vi "G#Object_UnregisterObject.vi"(0 "reference in":refnum<class "G#Object.lvclass">, 1 "object information":T1, 2 "object killed":bool, 3 "forced destroy":bool, 5 "error in (no error)":errorcluster) -> (14 "reference out":refnum<class "G#Object.lvclass">, 19 "error out":errorcluster)   [LabVIEW 2017, in "G#Object.lvclass"]
doc: "Unregisters the object from the G# object lists. It also sends an event to the debugger and desktop trace."
uses:
  G#Object.lvclass
  utils/G#Object_ObjectInfoType.ctl
  utils/G#Object_CreateMethod.ctl
  G#Object.lvclass/G#Object.ctl
  utils/G#Object_EventType.ctl
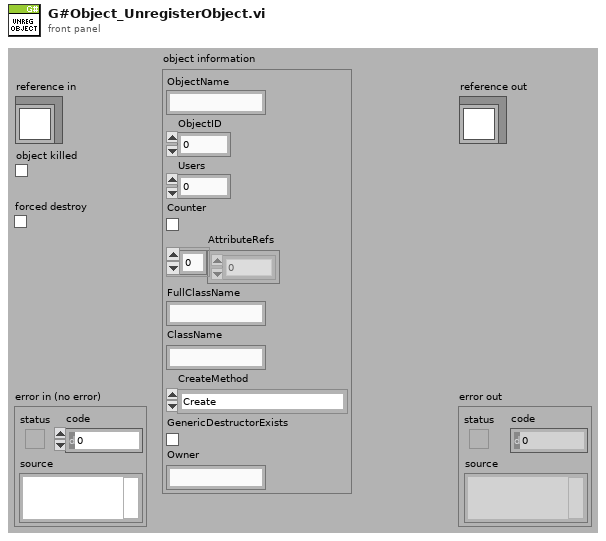
[diagram p1: front panel]
types:
  T1 = typedef "G#Object.lvclass/G#Object_ObjectInfoType.ctl" = cluster{"ObjectName":string, "ObjectID":u32, "Users":i32, "Counter":bool, "AttributeRefs":u32[], "FullClassName":string, "ClassName":string, "CreateMethod":T2, "GenericDestructorExists":bool, "Owner":string}
  T2 = typedef "G#Object.lvclass/G#Object_CreateMethod.ctl" = enum16{"Create", "Create or look up existing", "Look up existing"}
  T3 = typedef "G#Object.lvclass/G#Object_EventType.ctl" = enum16{"Created new", "Looked up existing", "Deleted", "Forced delete", "Not deleted", "Garbage collected", "Cleared", "User", "Error", "External create object", "External create class attributes", "Created class attributes", "Run constructor", "Run constructor done", "Run open method", "Run open method done"}
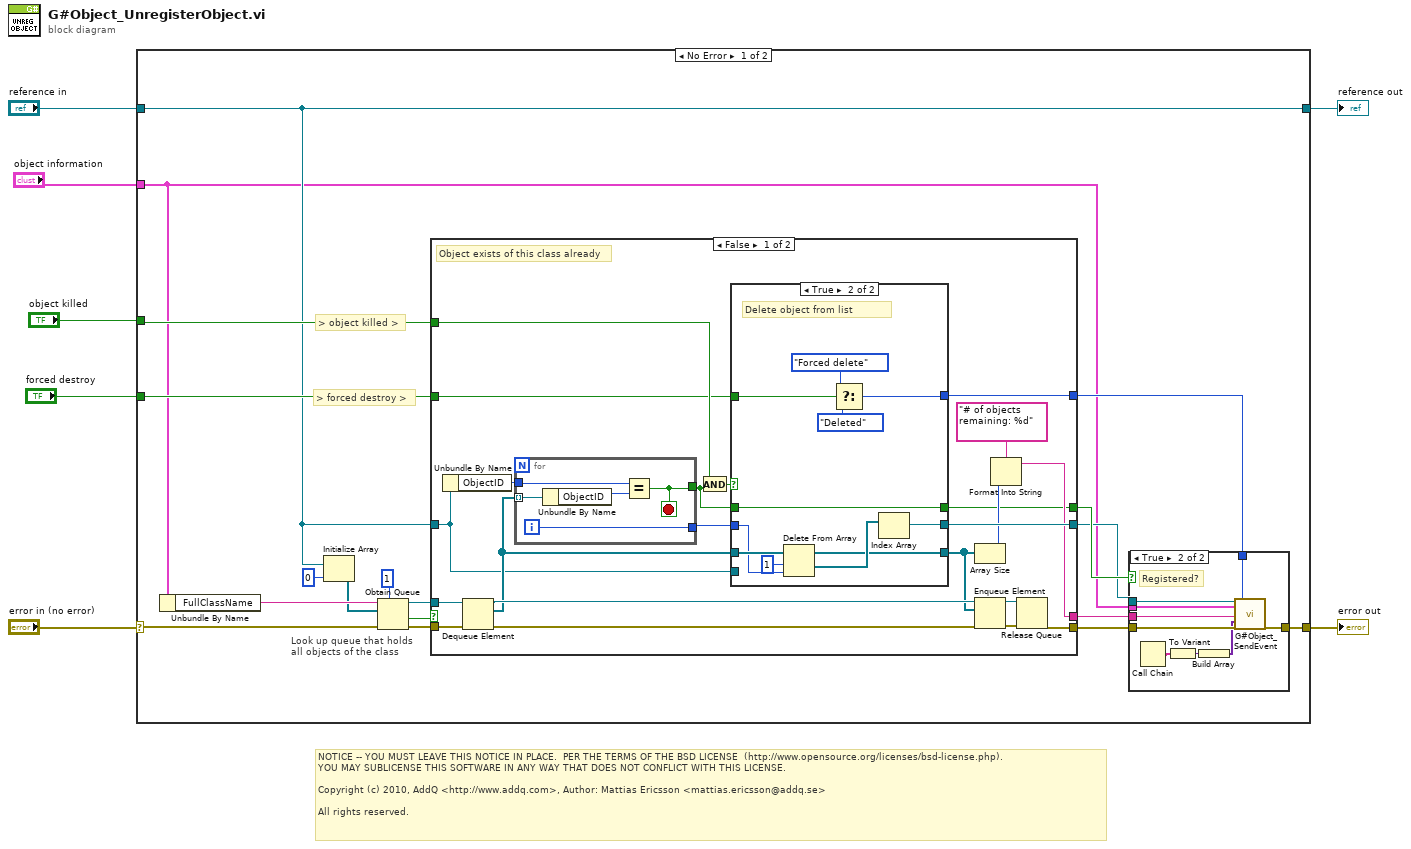
[diagram p0: block diagram]
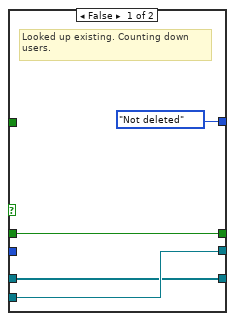
[diagram p3: hidden frame]
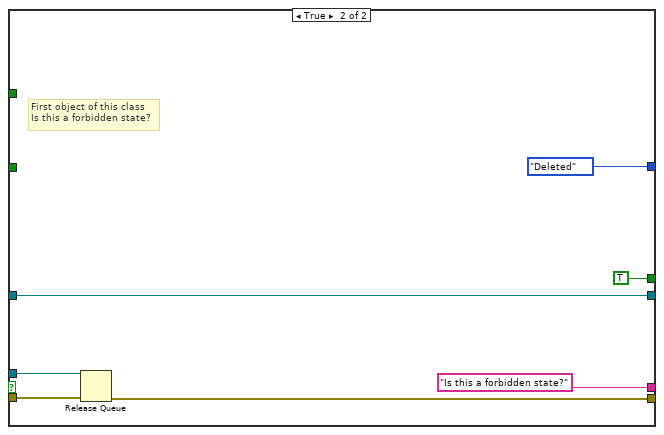
[diagram p4: hidden frame]
diagram:
  # "NOTICE -- YOU MUST LEAVE THIS NOTICE IN PLACE.  PER THE TERMS OF THE BSD LICENSE  (http://www.opensource.org/licenses/bsd-license.php).\nYOU MAY SUBLICENSE THIS SOFTWARE IN ANY WAY THAT DOES NOT CONFLICT WITH THIS LICENSE.\n\nCopyright (c) 2010, AddQ <http://www.addq.com>, Author: Mattias Ericsson <mattias.ericsson@addq.se>\n\nAll rights reserved."
  n1 = case shown="No Error" "error in (no error)" {
    selector: "error in (no error)" -> [w15 w86]
    tunnel: [w16 w86] -> w6
    tunnel: [w13 w85] -> w4
    tunnel: "reference in" -> [w13 w85]
    tunnel: "object killed" -> [w18 _]
    tunnel: "forced destroy" -> [w17 _]
    tunnel: "object information" -> [w8 _]
    frame No Error {
      # "> object killed >"
      # "> forced destroy >"
      # "Look up queue that holds\nall objects of the class"
      n2 = Unbundle By Name(w8) -> ("FullClassName"=w14:string)
      n3 = Initialize Array(w13, 0 ("dimension size")) -> (w11:refnum<class "G#Object.lvclass">[])
      n4 = Obtain Queue(max queue size (-1, unlimited)=1, name (unnamed)=w14, element data type=w11, error in (no error)=w15) -> (queue out=w22:refnum<queue>, created new?=w23:bool, error out=w24:errorcluster)  [unwired: 1 in]
      n5 = case shown="False" w23 {
        tunnel: w24 -> [w57 w84]
        tunnel: w22 -> [w56 w82]
        tunnel: [w53 w83] -> w21
        tunnel: w13 -> [w42 w81]
        tunnel: w18 -> [w48 _]
        tunnel: w17 -> [w47 _]
        tunnel: [w44 w81] -> w9
        tunnel: [w45 G#Object_EventType."Deleted" ("G#Event")] -> w20
        tunnel: [w38 "Is this a forbidden state?"] -> w19
        tunnel: [w36 TRUE] -> w10
        frame False {
          # "Object exists of this class already"
          n6 = Unbundle By Name(w42) -> ("ObjectID"=w43:u32)
          n7 = Dequeue Element(queue=w56, error in (no error)=w57) -> (queue out=w55:refnum<queue>, element=w50:refnum<class "G#Object.lvclass">[], error out=w54:errorcluster)  [unwired: 1 in, 1 out]
          n8 = for {
            tunnel: w50 -> [w77] mode=indexing
            tunnel: w43 -> [w75]
            tunnel: [w74] -> w46
            tunnel: [w73] -> w37
            i -> [w74]
            stop <- w73 stop-if-true
            n9 = Unbundle By Name(w77) -> ("ObjectID"=w76:u32)
            n10 = Equal?(x=w75, y=w76) -> (x = y?=w73:bool)
          }
          n11 = And(x=w48, y=w37) -> (x .and. y?=w49:bool)
          n12 = case shown="True" w49 {
            tunnel: w50 -> [w59 w72]
            tunnel: [w59 w63] -> w40
            tunnel: w47 -> [_ w70]
            tunnel: [w60 w65] -> w44
            tunnel: w46 -> [_ w66]
            tunnel: [G#Object_EventType."Not deleted" ("G#Event") w67] -> w45
            tunnel: w42 -> [w60 _]
            tunnel: w37 -> [w58 w62]
            tunnel: [w58 w62] -> w36
            frame False {
              # "Looked up existing. Counting down\nusers."
            }
            frame True {
              # "Delete object from list"
              n13 = Delete From Array(array=w72, length=1, index=w66) -> (deleted portion=w64:refnum<class "G#Object.lvclass">[], array with subset deleted=w63:refnum<class "G#Object.lvclass">[])
              n14 = Select(t=G#Object_EventType."Forced delete" ("G#Event"), s=w70, f=G#Object_EventType."Deleted" ("G#Event")) -> (s? t:f=w67:T3)
              n15 = Index Array(array=w64) -> (element=w65:refnum<class "G#Object.lvclass">)  [unwired: 1 in]
            }
          }
          n16 = Array Size(array=w40) -> (size(s)=w39:i32)
          n17 = Enqueue Element(queue=w55, element=w40, error in (no error)=w54) -> (queue out=w51:refnum<queue>, error out=w52:errorcluster)  [unwired: 1 in, 1 out]
          n18 = Format Into String(format string="# of objects remaining: %d", w39) -> (resulting string=w38:string)  [unwired: 2 in, 1 out]
          n19 = Release Queue(queue=w51, error in (no error)=w52) -> (error out=w53:errorcluster)  [unwired: 1 in, 2 out]
        }
        frame True {
          # "First object of this class\nIs this a forbidden state?"
          n20 = Release Queue(queue=w82, error in (no error)=w84) -> (error out=w83:errorcluster)  [unwired: 1 in, 2 out]
        }
      }
      n21 = case shown="True" w10 {
        tunnel: w21 -> [w26 w35]
        tunnel: w20 -> [_ w34]
        tunnel: w19 -> [_ w33]
        tunnel: [w26 w32] -> w16
        tunnel: w8 -> [_ w31]
        tunnel: w9 -> [_ w30]
        frame False {
        }
        frame True {
          # "Registered?"
          n22 = Call Chain() -> (call chain=w29:string[])
          n23 = To Variant(anything=w29) -> (Variant=w28:variant)
          n24 = Build Array(w28) -> (w27:variant[])
          n25 = call "G#Object_SendEvent.vi"("reference in"=w30, "object info extended"=w31, "comment"=w33, "parameters"=w27, "error in (no error)"=w35, "G# event type"=w34) -> ("error out"=w32:errorcluster)  [unwired: 13 in]
        }
      }
    }
    frame Error {
    }
  }
  "error out" <- w6
  "reference out" <- w4
